vi "Save_Tracking_Results_Movie-2.vi"(5 "Save movies":bool, 6 "FPS":u32, 7 "# codec":i32, 8 "error IN":errorcluster, 9 "AVI Refnum":T1, 10 "default name":string, 11 "(X,Y,dX,dY)":dbl[][](array[numeric])) -> (0 "error out":errorcluster)   [LabVIEW 2017]
uses:
  <vilib>/vision/Avi.llb/IMAQ AVI2 Refnum.ctl
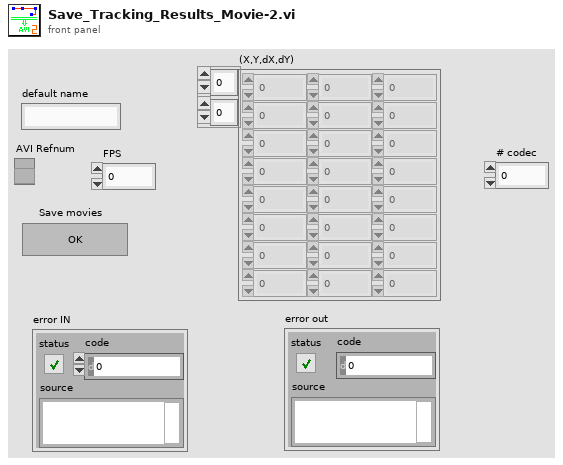
[diagram p1: front panel]
types:
  T1 = typedef "IMAQ AVI2 Refnum.ctl" = refnum<k20>
  T2 = typedef "Image Type" = u32
  T3 = typedef "IMAQ Image.ctl" = refnum<image>
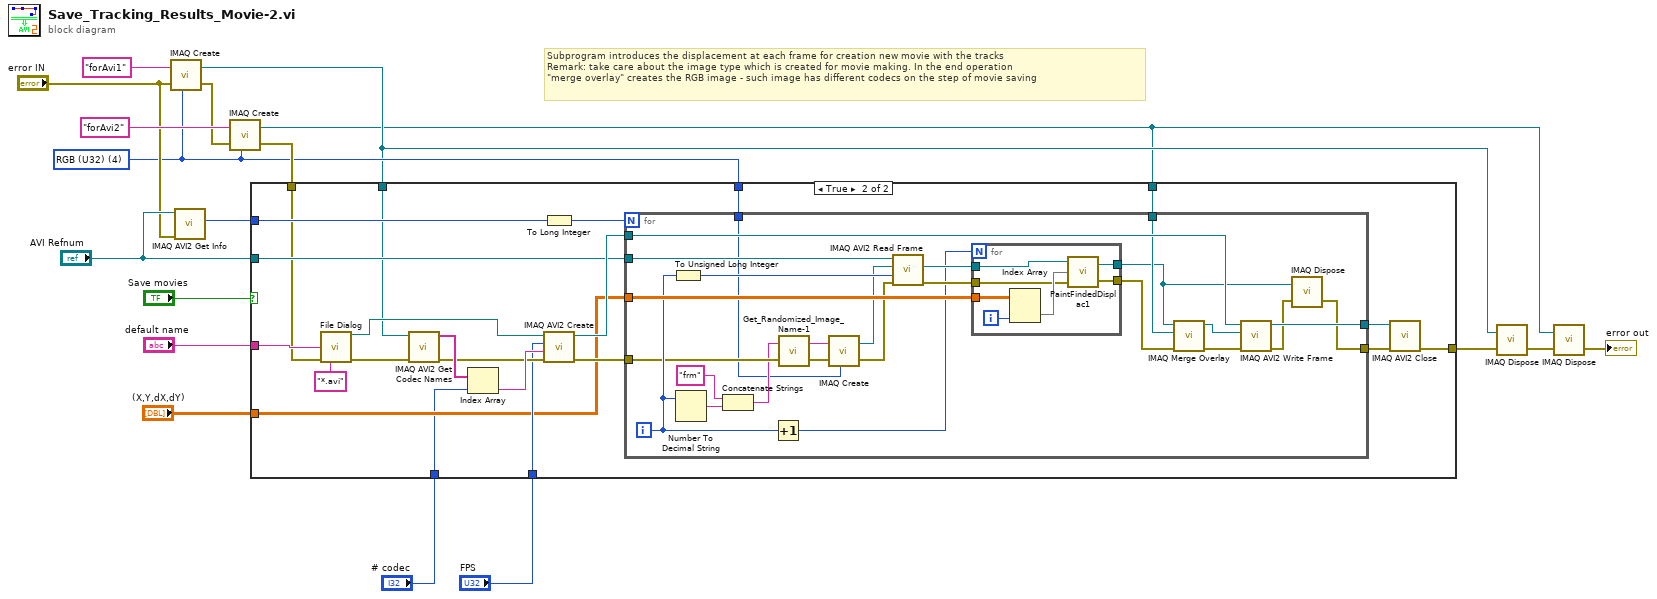
[diagram p0: block diagram]
diagram:
  w6 = T2 4 items=["Grayscale (U8)", "Grayscale (I16)", "Grayscale (SGL)", "Complex (CSG)", "RGB (U32)", "HSL (U32)", "RGB (U64)", "Grayscale (U16)"] ("Image Type")
  # "Subprogram introduces the displacement at each frame for creation new movie with the tracks\nRemark: take care about the image type which is created for movie making. In the end operation\n\"merge overlay\" creates the RGB image - such image has different codecs on the step of movie saving"
  n1 = call "IMAQ Create"("Image Name"="forAvi1", "Image Type"=w6, "error in (no error)"="error IN") -> ("New Image"=w4:T3, "error out"=w8:errorcluster)  [unwired: 2 in]
  n2 = call "IMAQ AVI2 Get Info"("error in (no error)"="error IN", "AVI Refnum"="AVI Refnum") -> ("Number of Frames"=w15:u32)  [unwired: 5 in, 4 out]
  n3 = call "IMAQ Create"("Image Name"="forAvi2", "Image Type"=w6, "error in (no error)"=w8) -> ("New Image"=w2:T3, "error out"=w7:errorcluster)  [unwired: 2 in]
  n4 = case shown="True" "Save movies" {
    tunnel: w15 -> [_ w29]
    tunnel: w4 -> [_ w22]
    tunnel: "FPS" -> [_ w34]
    tunnel: "(X,Y,dX,dY)" -> [_ w33]
    tunnel: "AVI Refnum" -> [_ w32]
    tunnel: [w19 w26] -> w5
    tunnel: "default name" -> [_ w30]
    tunnel: w7 -> [w19 w24]
    tunnel: "# codec" -> [_ w23]
    tunnel: w2 -> [_ w21]
    tunnel: w6 -> [_ w20]
    frame False {
    }
    frame True {
      n5 = call "File Dialog"("default name"=w30, "error in"=w24, "pattern (all files)"="*.avi") -> ("selected path"=w35:path, "error out"=w31:errorcluster)  [unwired: 9 in, 2 out]
      n6 = call "IMAQ AVI2 Get Codec Names"("error in (no error)"=w31, "Image"=w22) -> ("error out"=w39:errorcluster, "Codec Names"=w41:string[])  [unwired: 8 in]
      n7 = Index Array(array=w41, index=w23) -> (element=w40:string)
      n8 = To Long Integer(number=w29) -> (32bit integer=w28:i32)
      n9 = call "IMAQ AVI2 Create"("error in (no error)"=w39, "Codec"=w40, "Frames Per Second"=w34, "AVI Path"=w35) -> ("error out"=w38:errorcluster, "AVI Refnum"=w37:T1)  [unwired: 6 in]
      n10 = for {
        N: w28 -> [_]
        tunnel: w32 -> [w66]
        tunnel: w38 -> [w52]
        tunnel: w37 -> [w65]
        tunnel: w33 -> [w60]
        tunnel: [w42] -> w27
        tunnel: [w62] -> w25
        tunnel: w21 -> [w61]
        tunnel: w20 -> [w48]
        i -> [w54]
        n11 = To Unsigned Long Integer(number=w54) -> (unsigned 32bit integer=w53:u32)
        n12 = Number To Decimal String(number=w54) -> (decimal integer string=w56:string)  [unwired: 1 in]
        n13 = Concatenate Strings("frm" ("string"), w56) -> (w51:string)
        n14 = Increment(x=w54) -> (x+1=w45:i32)
        n15 = call "Get_Randomized_Image_Name-1.vi"("error IN"=w52, "Main Name"=w51) -> ("error OUT"=w49:errorcluster, "Randomized name"=w50:string)
        n16 = call "IMAQ Create"("Image Name"=w50, "Image Type"=w48, "error in (no error)"=w49) -> ("New Image"=w47:T3, "error out"=w46:errorcluster)  [unwired: 2 in]
        n17 = call "IMAQ AVI2 Read Frame"("error in (no error)"=w46, "Frame Number"=w53, "Image"=w47, "AVI Refnum"=w66) -> ("error out"=w59:errorcluster, "Image Out"=w58:T3)  [unwired: 5 in, 1 out]
        n18 = for {
          N: w45 -> [_]
          tunnel: w60 -> [w73]
          tunnel: w59 -> [w69]
          tunnel: w58 -> [w70]
          tunnel: [w68] -> w44
          tunnel: [w67] -> w57
          i -> [w72]
          n19 = Index Array(array=w73, index (col)=w72) -> (element=w71:dbl[])  [unwired: 1 in]
          n20 = call "PaintFindedDisplac1.vi"("error IN"=w69, "Array of Points IN"=w71, "Image IN"=w70) -> ("error OUT"=w67:errorcluster, "Image OUT"=w68:T3)
        }
        n21 = call "IMAQ Merge Overlay"("error in (no error)"=w57, "Image Dst"=w61, "Image Src"=w44) -> ("error out"=w63:errorcluster, "Image Dst Out"=w64:T3)  [unwired: 7 in]
        n22 = call "IMAQ AVI2 Write Frame"("error in (no error)"=w63, "Image"=w64, "AVI Refnum"=w65) -> ("error out"=w43:errorcluster, "AVI Refnum (duplicate)"=w62:T1)  [unwired: 6 in, 1 out]
        n23 = call "IMAQ Dispose"("Image"=w44, "error in (no error)"=w43) -> ("error out"=w42:errorcluster)  [unwired: 4 in]
      }
      n24 = call "IMAQ AVI2 Close"("error in (no error)"=w27, "AVI Refnum"=w25) -> ("error out"=w26:errorcluster)  [unwired: 9 in]
    }
  }
  n25 = call "IMAQ Dispose"("Image"=w4, "error in (no error)"=w5) -> ("error out"=w3:errorcluster)  [unwired: 4 in]
  n26 = call "IMAQ Dispose"("Image"=w2, "error in (no error)"=w3) -> ("error out"=→"error out":errorcluster)  [unwired: 4 in]
